vi "2nd_Order_Roots.vi"(4 "data":variant, 5 "X":dbl[](array[numeric])) -> (2 "F(X)":dbl[](array[numeric]))   [LabVIEW 2012]
uses:
  2nd_Order_TD.ctl
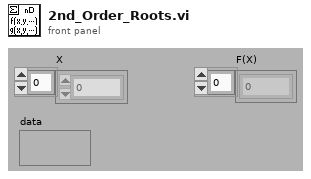
[diagram p1: front panel]
types:
  T1 = typedef "2nd_Order_TD.ctl" = cluster{"omega_h":dbl, "zeta":dbl, "omega":dbl}
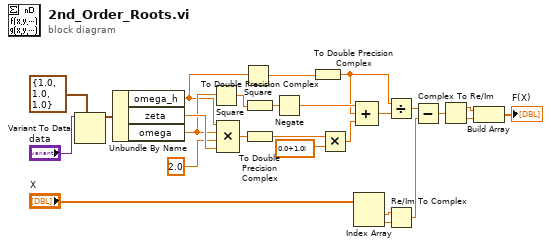
[diagram p0: block diagram]
diagram:
  n1 = Variant To Data(type=T1 {"omega_h"=1.0, "zeta"=1.0, "omega"=1.0} ("2nd Oder TD"), Variant="data") -> (data=w25:T1)  [unwired: 1 in, 1 out]
  n2 = Unbundle By Name(w25) -> ("omega_h"=w14:dbl, "zeta"=w24:dbl, "omega"=w15:dbl)
  n3 = Square(x=w15) -> (x^2=w7:dbl)
  n4 = Compound Arithmetic op=MULTIPLY(w14, w15, 2.0 ("value"), w24) -> (w9:dbl)
  n5 = Square(x=w14) -> (x^2=w4:dbl)
  n6 = To Double Precision Complex(1:w7) -> (0:w6:cdb)
  n7 = To Double Precision Complex(1:w9) -> (0:w10:cdb)
  n8 = Negate(x=w6) -> (-x=w8:cdb)
  n9 = To Double Precision Complex(1:w4) -> (0:w5:cdb)
  n10 = Multiply(x=w10, y=cdb 0.0+1.0i) -> (x*y=w12:cdb)
  n11 = Index Array(array="X") -> (element #1=w18:dbl, element #2=w17:dbl)  [unwired: 2 in]
  n12 = Compound Arithmetic op=ADD(w8, w5, w12) -> (w2:cdb)
  n13 = Divide(x=w5, y=w2) -> (x/y=w1:cdb)
  n14 = Re/Im To Complex(1:w17, 2:w18) -> (0:w16:cdb)
  n15 = Subtract(x=w1, y=w16) -> (x-y=w13:cdb)
  n16 = Complex To Re/Im(x + iy=w13) -> (x=w21:dbl, y=w20:dbl)
  n17 = Build Array(w21, w20) -> (→"F(X)":dbl[])
